vi "INTELLIFAUCET MicroAmp Set.vi"(4 "Refnum in":T1, 5 "milliseconds to wait":u32=100, 6 "Debug":bool, 7 "TEMP,FLOW":T2=enum."FLOW", 8 "error in (no error)":errorcluster, 9 "# of Retries":i32=1, 10 "MicroAmp":i32, 11 "VISA Refnum in":refnum<visa-resource-name>) -> (0 "error out":errorcluster, 3 "VISA Refnum out":refnum<visa-resource-name>)   [LabVIEW 2016]
uses:
  Type Definitions/INTELLIFAUCT Temp Flow.ctl
  MW100/Type Definitions/HEWH MW100 Channel Numbers.ctl
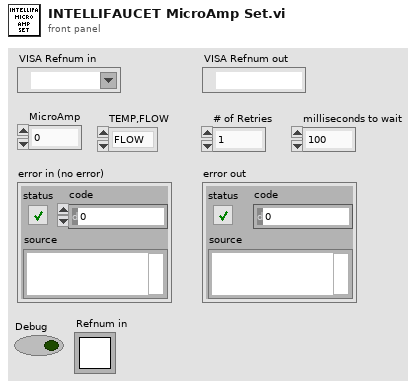
[diagram p1: front panel]
types:
  T1 = typedef "Semaphore RefNum" = refnum<k1>
  T2 = typedef "INTELLIFAUCT Temp Flow.ctl" = enum8{"TEMP", "FLOW"}
  T3 = typedef "HEWH MW100 Channel Numbers.ctl" = string
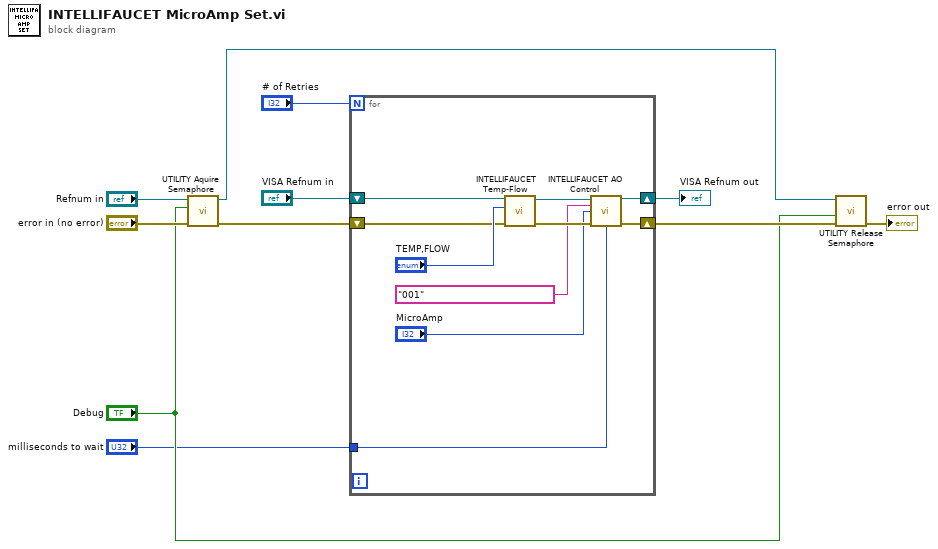
[diagram p0: block diagram]
diagram:
  n1 = call "UTILITY Aquire Semaphore.vi"("error in (no error)"="error in (no error)", "Debug"="Debug", "Refnum in"="Refnum in") -> ("error out"=w5:errorcluster, "Refnum out"=w3:T1)  [unwired: 6 in, 1 out]
  n2 = for {
    N: "# of Retries" -> [_]
    shift-right: [w15] -> w8
    shift-left: w5 -> [w14]
    shift-right: [w16] -> w10
    shift-left: "VISA Refnum in" -> [w18]
    tunnel: "milliseconds to wait" -> [w12]
    n3 = call "INTELLIFAUCET Temp-Flow.vi"("Error In"=w14, "TEMP,FLOW"="TEMP,FLOW", "VISA session"=w18) -> ("Error Out"=w20:errorcluster, "dup VISA session"=w17:refnum<visa-resource-name>)  [unwired: 7 in]
    n4 = call "INTELLIFAUCET AO Control.vi"("VISA session"=w17, "HEWH MW100 Channel Numbers"=T3 "001", "Output Value (0)"="MicroAmp", "Error In"=w20, "milliseconds to wait"=w12) -> ("dup VISA session"=w16:refnum<visa-resource-name>, "error out"=w15:errorcluster)  [unwired: 9 in]
  }
  "VISA Refnum out" <- w10
  n5 = call "UTILITY Release Semaphore.vi"("error in (no error)"=w8, "Debug"="Debug", "Refnum in"=w3) -> ("error out"=→"error out":errorcluster)  [unwired: 8 in]
